vi "Calculate Target Pose.vi"(6 "Distance to target (in)":dbl=36.0, 8 "Robot Calibration Cluster":T1={"Camera Height on robot (in)"=34.5, "Camera Angle on the robot (deg)"=28.3, "Camera FOV Top to Bottom View Angle (deg)"=0.946, "Camera FOV Left to Right View Angle (deg)"=26.5, "Target size (in)"=6.5, "Distance to front of bumper (in)"=9.75, "Focal Length (mm)"=10.0, "Yaw Slope"=9.75, "Yaw Offset"=10.0} {"Yaw Offset" format="%#_13g"; "Yaw Slope" format="%#_13g"; "Camera FOV Left to Right View Angle (deg)" format="%#_13g"; "Focal Length (mm)" format="%#_13g"; "Distance to front of bumper (in)" format="%#_13g"; "Target size (in)" format="%#_13g"; "Camera FOV Top to Bottom View Angle (deg)" format="%#_13g"; "Camera Angle on the robot (deg)" format="%#_13g"; "Camera Height on robot (in)" format="%#_13g"}, 9 "Camera Resolution":T2={"Camera Resolution W (pixels)"=800.0, "Camera Resolution H (pixels)"=600.0}, 10 "Corners":cluster{"X":dbl, "Y":dbl}[](array[cluster])=[{"X"=420.0, "Y"=290.0}, {"X"=480.0, "Y"=290.0}, {"X"=420.0, "Y"=350.0}, {"X"=480.0, "Y"=350.0}], 11 "Target Center":cluster{"X":dbl, "Y":dbl}) -> (1 "Target Roll (deg)":dbl, 2 "Target Pitch (deg)":dbl, 3 "Target Yaw (deg)":dbl)   [LabVIEW 2023]
uses:
  Camera Info.ctl
panel:
  out "3D Position (inches)":cluster{"X":dbl, "Y":dbl, "Z":dbl}
  out "Z'":dbl
  out "Y'":dbl
  out "Z (in)":dbl=36.0
  out "Y (in)":dbl
  out "X (in)":dbl
  out "Theta y (deg)":dbl
  out "Theta x (deg)":dbl
  out "Focal length in pixels":dbl
  out "Sensor height (mm)":dbl
  out "Sensor width (mm)":dbl
  in  "Sensor pixel size (µm)":dbl=3.0
  # "Bottom Left"
  # "Bottom Right"
  # "Top Right"
  # "Top Left"
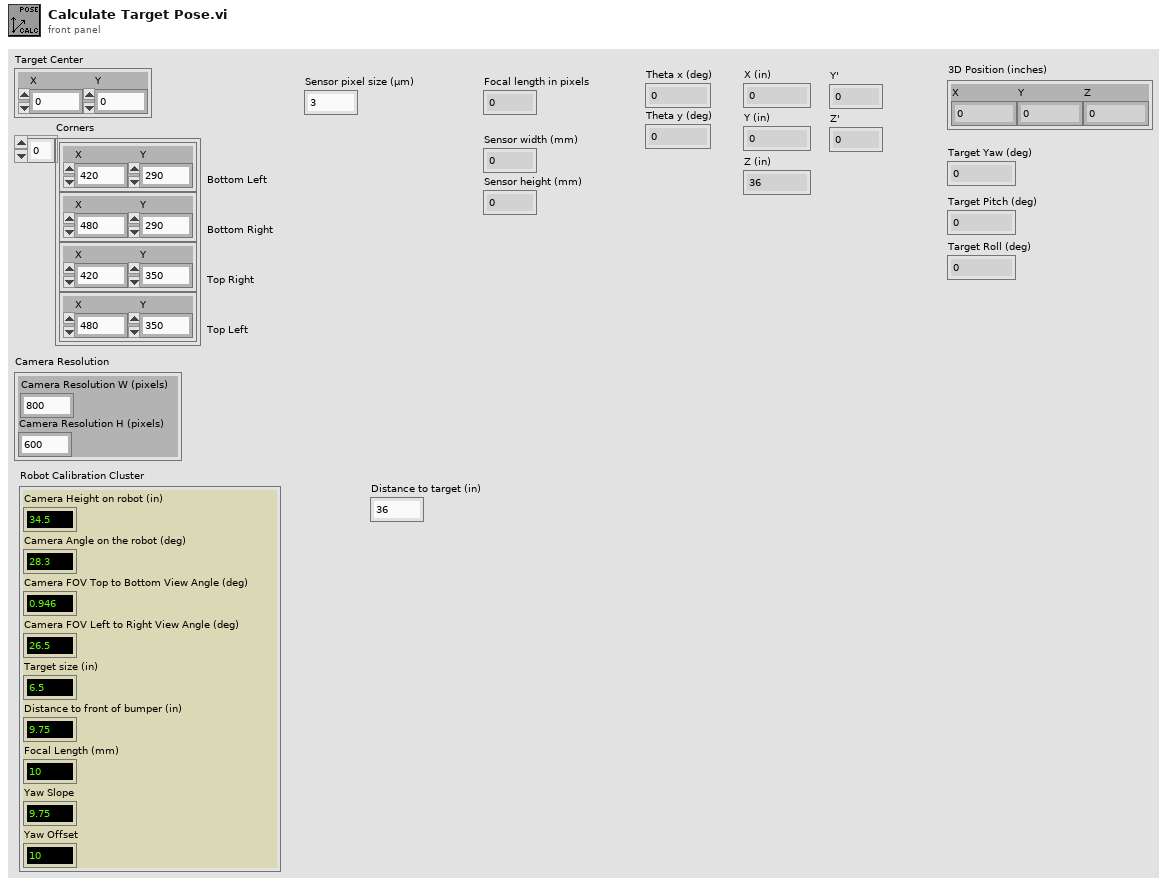
[diagram p1: front panel]
types:
  T1 = typedef "Camera Info.ctl" = cluster{"Camera Height on robot (in)":dbl, "Camera Angle on the robot (deg)":dbl, "Camera FOV Top to Bottom View Angle (deg)":dbl, "Camera FOV Left to Right View Angle (deg)":dbl, "Target size (in)":dbl, "Distance to front of bumper (in)":dbl, "Focal Length (mm)":dbl, "Yaw Slope":dbl, "Yaw Offset":dbl}
  T2 = cluster{"Camera Resolution W (pixels)":dbl, "Camera Resolution H (pixels)":dbl}
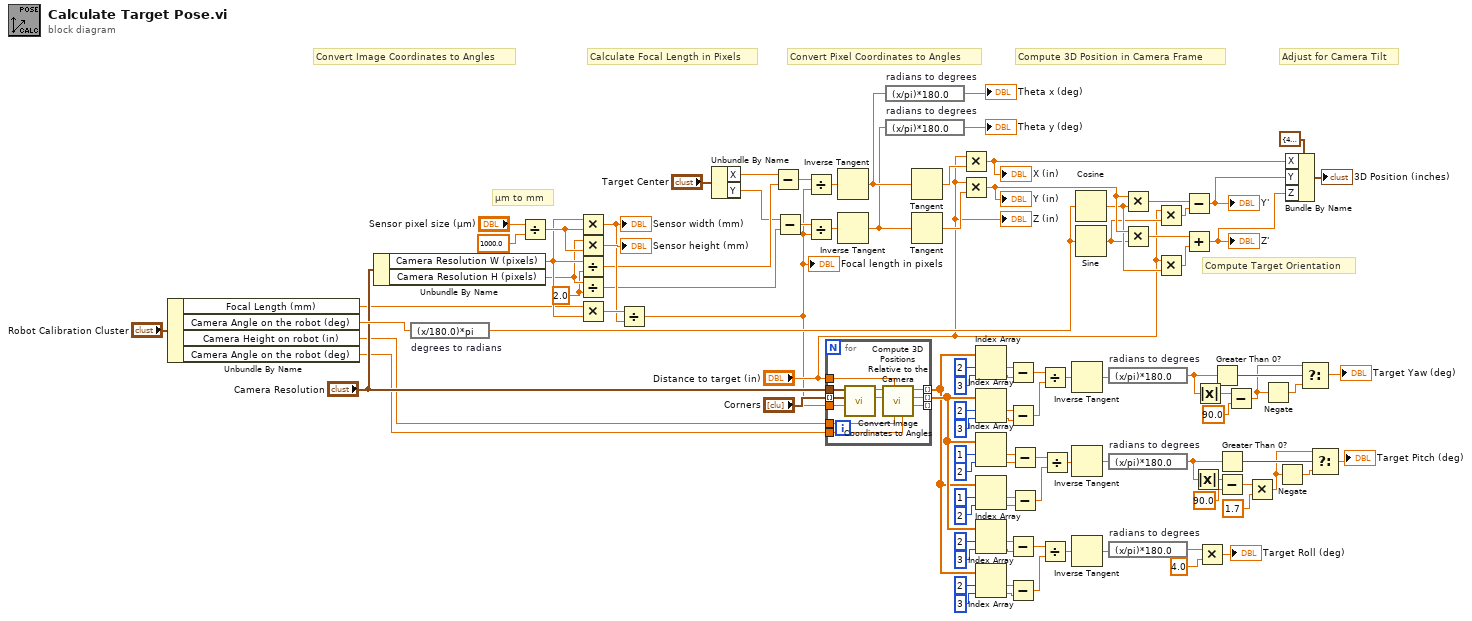
[diagram p0: block diagram]
diagram:
  w72 = 2.0 ("y")
  # "Compute Target Orientation"
  # "Adjust for Camera Tilt"
  # "Compute 3D Position in Camera Frame"
  # "Convert Pixel Coordinates to Angles"
  # "Calculate Focal Length in Pixels"
  # "µm to mm"
  # "Convert Image Coordinates to Angles"
  n1 = Unbundle By Name("Robot Calibration Cluster") -> ("Focal Length (mm)"=w24:dbl, "Camera Angle on the robot (deg)"=w68:dbl, "Camera Height on robot (in)"=w61:dbl, "Camera Angle on the robot (deg)"=w60:dbl)
  n2 = Unbundle By Name("Camera Resolution") -> ("Camera Resolution W (pixels)"=w74:dbl, "Camera Resolution H (pixels)"=w73:dbl)
  n3 = expression code="(x/180.0)*pi" "degrees to radians"(w68) -> (w80:dbl)
  n4 = Divide(x="Sensor pixel size (µm)", y=1000.0) -> (x/y=w101:dbl)
  n5 = Multiply(x=w74, y=w101) -> (x*y=w98:dbl)
  "Sensor width (mm)" <- w98
  n6 = Multiply(x=w73, y=w101) -> (x*y=→"Sensor height (mm)":dbl)
  n7 = Divide(x=w74, y=w72) -> (x/y=w71:dbl)
  n8 = Divide(x=w73, y=w72) -> (x/y=w70:dbl)
  n9 = Multiply(x=w24, y=w74) -> (x*y=w99:dbl)
  n10 = Divide(x=w99, y=w98) -> (x/y=w23:dbl)
  "Focal length in pixels" <- w23
  n11 = Unbundle By Name("Target Center") -> ("X"=w66:dbl, "Y"=w65:dbl)
  n12 = Subtract(x=w66, y=w71) -> (x-y=w97:dbl)
  n13 = Subtract(x=w65, y=w70) -> (x-y=w96:dbl)
  n14 = Divide(x=w97, y=w23) -> (x/y=w95:dbl)
  n15 = Divide(x=w96, y=w23) -> (x/y=w94:dbl)
  n16 = for {
    tunnel: "Camera Resolution" -> [w114]
    tunnel: w23 -> [w113]
    tunnel: "Corners" -> [w112] mode=indexing
    tunnel: "Distance to target (in)" -> [w111]
    tunnel: [w110] -> w21 mode=indexing
    tunnel: [w109] -> w22 mode=indexing
    tunnel: [w108] -> _ mode=indexing
    tunnel: w61 -> [w107]
    tunnel: w60 -> [w106]
    n17 = call "Convert Image Coordinates to Angles.vi"("Focal length in pixels"=w113, "Corner"=w112, "Camera Resolution"=w114) -> ("Theta Y"=w104:dbl, "Theta Z"=w105:dbl)  [unwired: 7 in]
    n18 = call "Compute 3D Positions Relative to the Camera.vi"("Camera Angle on the robot (deg)"=w106, "Camera Height on robot (in)"=w107, "Distance to target (in)"=w111, "Thata Y"=w104, "Thata Z"=w105) -> ("Z Corrected"=w108:dbl, "Y Corrected"=w109:dbl, "X (in)"=w110:dbl)  [unwired: 4 in]
  }
  n19 = Inverse Tangent(1:w95) -> (0:w89:dbl)
  n20 = Inverse Tangent(1:w94) -> (0:w88:dbl)
  n21 = expression code="(x/pi)*180.0" "radians to degrees"(w89) -> (→"Theta x (deg)":dbl)
  n22 = expression code="(x/pi)*180.0" "radians to degrees"(w88) -> (→"Theta y (deg)":dbl)
  n23 = Tangent(1:w89) -> (0:w92:dbl)
  n24 = Tangent(1:w88) -> (0:w90:dbl)
  n25 = Multiply(x="Distance to target (in)", y=w92) -> (x*y=w77:dbl)
  "X (in)" <- w77
  n26 = Multiply(x="Distance to target (in)", y=w90) -> (x*y=w87:dbl)
  "Y (in)" <- w87
  n27 = Index Array(array=w21, index #1=2 ("index"), index #2=3 ("index")) -> (element #1=w57:dbl, element #2=w56:dbl)
  n28 = Index Array(array=w22, index #1=2 ("index"), index #2=3 ("index")) -> (element #1=w54:dbl, element #2=w55:dbl)
  n29 = Index Array(array=w22, index #1=1 ("index"), index #2=2 ("index")) -> (element #1=w15:dbl, element #2=w14:dbl)
  n30 = Index Array(array=w21, index #1=1 ("index"), index #2=2 ("index")) -> (element #1=w13:dbl, element #2=w12:dbl)
  n31 = Index Array(array=w22, index #1=2 ("index"), index #2=3 ("index")) -> (element #1=w44:dbl, element #2=w43:dbl)
  n32 = Index Array(array=w21, index #1=2 ("index"), index #2=3 ("index")) -> (element #1=w41:dbl, element #2=w42:dbl)
  n33 = Subtract(x=w57, y=w56) -> (x-y=w51:dbl)
  n34 = Subtract(x=w54, y=w55) -> (x-y=w50:dbl)
  n35 = Subtract(x=w44, y=w43) -> (x-y=w38:dbl)
  n36 = Subtract(x=w41, y=w42) -> (x-y=w37:dbl)
  n37 = Subtract(x=w15, y=w14) -> (x-y=w17:dbl)
  n38 = Subtract(x=w13, y=w12) -> (x-y=w18:dbl)
  n39 = Divide(x=w51, y=w50) -> (x/y=w49:dbl)
  n40 = Divide(x=w38, y=w37) -> (x/y=w36:dbl)
  n41 = Divide(x=w17, y=w18) -> (x/y=w16:dbl)
  n42 = Inverse Tangent(1:w49) -> (0:w48:dbl)
  n43 = Inverse Tangent(1:w16) -> (0:w19:dbl)
  n44 = Inverse Tangent(1:w36) -> (0:w35:dbl)
  n45 = Cosine(x=w80) -> (cos(x)=w82:dbl)
  n46 = Sine(x=w80) -> (sin(x)=w81:dbl)
  n47 = expression code="(x/pi)*180.0" "radians to degrees"(w48) -> (w29:dbl)
  n48 = expression code="(x/pi)*180.0" "radians to degrees"(w19) -> (w7:dbl)
  n49 = expression code="(x/pi)*180.0" "radians to degrees"(w35) -> (w33:dbl)
  n50 = Multiply(x=w87, y=w82) -> (x*y=w86:dbl)
  n51 = Multiply(x=w87, y=w81) -> (x*y=w84:dbl)
  n52 = Multiply(x="Distance to target (in)", y=w81) -> (x*y=w85:dbl)
  n53 = Multiply(x="Distance to target (in)", y=w82) -> (x*y=w83:dbl)
  n54 = Subtract(x=w86, y=w85) -> (x-y=w76:dbl)
  "Y'" <- w76
  n55 = Add(x=w84, y=w83) -> (x+y=w75:dbl)
  "Z'" <- w75
  n56 = Absolute Value(x=w7) -> (abs(x)=w9:dbl)
  n57 = Absolute Value(x=w29) -> (abs(x)=w30:dbl)
  n58 = Multiply(x=w33, y=4.0) -> (x*y=→"Target Roll (deg)":dbl)
  n59 = Greater Than 0?(x=w29) -> (x > 0?=w28:bool)
  n60 = Greater Than 0?(x=w7) -> (x > 0?=w10:bool)
  n61 = Subtract(x=w9, y=90.0) -> (x-y=w4:dbl)
  n62 = Subtract(x=w30, y=90.0) -> (x-y=w27:dbl)
  n63 = Multiply(x=w4, y=1.7) -> (x*y=w5:dbl)
  n64 = Negate(x=w27) -> (-x=w26:dbl)
  n65 = Negate(x=w5) -> (-x=w11:dbl)
  n66 = Bundle By Name(cluster=cluster{"X":dbl, "Y":dbl, "Z":dbl} {"X"=420.0, "Y"=290.0, "Z"=0.0} ("3D Position (inches)"), "X"=w77, "Y"=w76, "Z"=w75) -> (→"3D Position (inches)":cluster{"X":dbl, "Y":dbl, "Z":dbl})
  n67 = Select(t=w27, s=w28, f=w26) -> (s? t:f=→"Target Yaw (deg)":dbl)
  n68 = Select(t=w5, s=w10, f=w11) -> (s? t:f=→"Target Pitch (deg)":dbl)
  "Z (in)" <- "Distance to target (in)"
